vi "Write String.vi"(8 "Error In":errorcluster, 10 "Pair":cluster{"Key":string, "Value":string}, 11 "Data In":refnum<class "Data.lvclass">) -> (0 "Error Out":errorcluster, 3 "Data Out":refnum<class "Data.lvclass">)   [LabVIEW 2018, in "Toolkit.lvlib" / "Loaders.lvlib" / "Data.lvclass"]
doc: "Sets the key-value pair for a Partial tag where the Mustache partial template is stored in a string.\n\n<B>Data In/Out</B> - Represents a partial loader that loads partial Mustache templates either from a file if the value data type is a path or from memory if the value data type is a string.\n\n<B>Pair</B> - A key-value pair where the value is a string to a Mustache partial template stored in memory."
uses:
  Data.lvclass
  Data.lvclass/Data.ctl
  Data/String/String.lvclass
  D:/Users/cfield/Code/Field R&D Services/Labstache/src/Toolkit/Data/Datum/Datum.lvclass
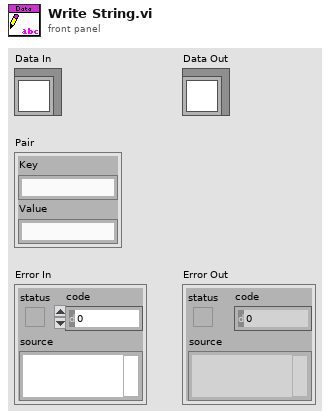
[diagram p1: front panel]
types:
  T1 = cluster{"Key":string, "Value":refnum<class "Datum.lvclass">}[]
  T2 = cluster{"Key":string, "String":refnum<class "String.lvclass">}
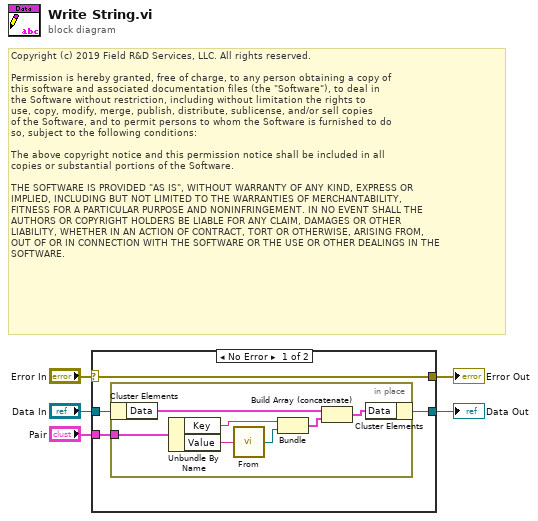
[diagram p0: block diagram]
diagram:
  # "Copyright (c) 2019 Field R&D Services, LLC. All rights reserved.\n\nPermission is hereby granted, free of charge, to any person obtaining a copy of\nthis software and associated documentation files (the \"Software\"), to deal in\nthe Software without restriction, including without limitation the rights to\nuse, copy, modify, merge, publish, distribute, sublicense, and/or sell copies\nof the Software, and to permit persons to whom the Software is furnished to do\nso, subject to the following conditions:\n\nThe above copyright notice and this permission notice shall be included in all\ncopies or substantial portions of the Software.\n\nTHE SOFTWARE IS PROVIDED \"AS IS\", WITHOUT WARRANTY OF ANY KIND, EXPRESS OR\nIMPLIED, INCLUDING BUT NOT LIMITED TO THE WARRANTIES OF MERCHANTABILITY,\nFITNESS FOR A PARTICULAR PURPOSE AND NONINFRINGEMENT. IN NO EVENT SHALL THE\nAUTHORS OR COPYRIGHT HOLDERS BE LIABLE FOR ANY CLAIM, DAMAGES OR OTHER\nLIABILITY, WHETHER IN AN ACTION OF CONTRACT, TORT OR OTHERWISE, ARISING FROM,\nOUT OF OR IN CONNECTION WITH THE SOFTWARE OR THE USE OR OTHER DEALINGS IN THE\nSOFTWARE."
  n1 = case shown="No Error" "Error In" {
    selector: "Error In" -> [w9 w18]
    tunnel: [w9 w18] -> w4
    tunnel: [w7 w17] -> w2
    tunnel: "Data In" -> [w8 w17]
    tunnel: "Pair" -> [w6 _]
    frame No Error {
      n2 = in-place {
        in-place-border: w6 -> [w14]
        n3 = in-place-cluster #1(w8) -> ("Data"=w16:T1)
        n4 = Unbundle By Name(w14) -> ("Key"=w13:string, "Value"=w11:string)
        n5 = call "From.vi"("Value"=w11) -> ("String"=w10:refnum<class "String.lvclass">)
        n6 = Bundle("Key"=w13, "String"=w10) -> (w12:T2)  [unwired: 1 in]
        n7 = Build Array (concatenate)(w16, w12) -> (w15:T1)
        n8 = in-place-cluster #1("Data"=w15) -> (w7:refnum<class "Data.lvclass">)
      }
    }
    frame Error {
    }
  }
  "Error Out" <- w4
  "Data Out" <- w2
